vi "Create Delimiter Object.vi"(7 "Delimiter in":refnum<class "Delimiter.lvclass">, 10 "Other":string, 11 "Delimiter":T1) -> (3 "Delimiter":refnum<class "Delimiter.lvclass">)   [LabVIEW 2014, in "Delimiter.lvclass"]
uses:
  Delimiter.lvclass
  Delimiters List.ctl
  Delimiter.lvclass/Delimiter.ctl
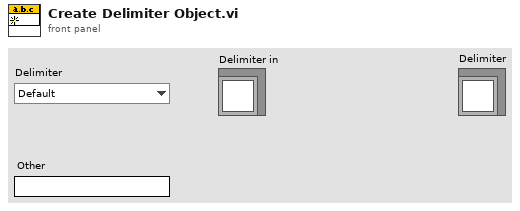
[diagram p1: front panel]
types:
  T1 = typedef "Delimiter.lvclass/Delimiters List.ctl" = enum16{"Default", "dot (.)", "colon (:)", "double-colon (::)", "semi-colon (;)", "underscore (_)", "double underscore (__)", "dash (-)", "double dash (--)", "backslash (\\)", "vertical bar (|)", "forward slash (/)", "chevron (>)", "double-chevron (>>)", "arrow (->)", "comma (,)", "arobas (@)", "ampersand (&)", "other"}
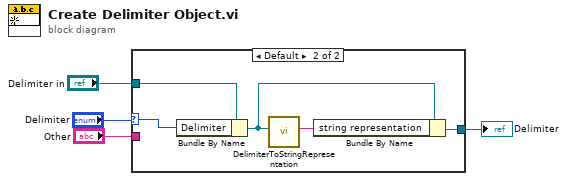
[diagram p0: block diagram]
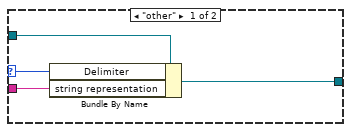
[diagram p2: hidden frame]
diagram:
  n1 = case shown="Default" "Delimiter" {
    selector: "Delimiter" -> [w7 w12]
    tunnel: "Delimiter in" -> [w8 w13]
    tunnel: "Other" -> [w6 _]
    tunnel: [w5 w11] -> w1
    frame "other" {
      n2 = Bundle By Name(cluster=w8, "Delimiter"=w7, "string representation"=w6) -> (w5:refnum<class "Delimiter.lvclass">)
    }
    frame Default {
      n3 = Bundle By Name(cluster=w13, "Delimiter"=w12) -> (w9:refnum<class "Delimiter.lvclass">)
      n4 = call "DelimiterToStringRepresentation.vi"("Delimiter"=w9) -> ("String representation"=w10:string)  [unwired: 10 in]
      n5 = Bundle By Name(cluster=w9, "string representation"=w10) -> (w11:refnum<class "Delimiter.lvclass">)
    }
  }
  "Delimiter" <- w1
